vi "JLINKARM Set Reset Type.vi"(8 "error in (no error)":errorcluster caption="错误输入（无错误）", 11 "ResetType":u32) -> (0 "error out":errorcluster caption="错误输出", 3 "function return":i32)   [LabVIEW 2016, in "JLinkARM.lvlib"]
doc: "int JLINKARM_SetResetType(unsigned long ResetType);"
uses:
  <userlib>/LV-JLinkARM/JLinkARM.lvlib
  <userlib>/LV-JLinkARM/JLinkARM.dll
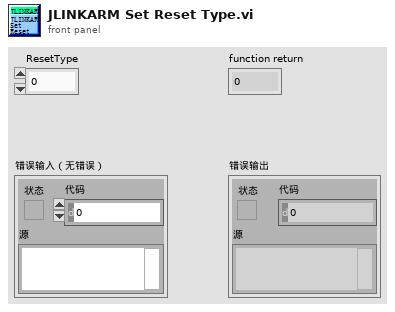
[diagram p1: front panel]
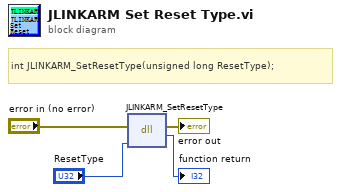
[diagram p0: block diagram]
diagram:
  # "int JLINKARM_SetResetType(unsigned long ResetType);"
  n1 = dll-call lib="C:/Program Files (x86)/National Instruments/LabVIEW 2016/user.lib/LV-JLinkARM/JLinkARM.*" fn="JLINKARM_SetResetType"(error in="error in (no error)", "ResetType"="ResetType") -> (error out=→"error out":errorcluster, →"function return":i32)  [unwired: 3 in, 1 out]
